vi "Read Swipe Vector.vi"   [LabVIEW 2011, in "LVH-Leap.lvlib"]
doc: "Read swipe gesture vectors. Use the polymorphic instance to select between one and N swipe gestures."
uses:
  LVH-Leap.lvlib
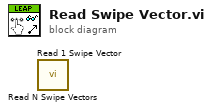
[diagram p0: block diagram]
diagram:
  n1 = call "Read N Swipe Vectors.vi"() -> ()  [unwired: 8 in, 4 out]
  n2 = call "Read 1 Swipe Vector.vi"() -> ()  [unwired: 8 in, 4 out]
